vi "ramp autonomous.vi"() -> ()   [LabVIEW 2012, in "Omni2013.lvrbt"]
uses:
  Omni2013.lvrbt
  <vilib>/NXT/Hardware/Plugins/Tetrix 180 deg Servo/Tetrix180ServoAddress.ctl
  <vilib>/NXT/Hardware/Plugins/Tetrix DC Motor/TetrixDCMotorAddress.ctl
  <vilib>/NXT/HiTechnic/HiTechnic Controls/HiTechnic Port.ctl
  <vilib>/NXT/Block Support/NXT_InputPort.ctl
  <vilib>/NXT/Dual Mode Library/Waits/Wait_Num(msec).vi
  <vilib>/NXT/NXTIO Xnodes/NXTIONodeSubVIs/TETRIX IO Move Servos.vi
  <vilib>/NXT/NXTIO Xnodes/NXTIONodeSubVIs/TETRIX IO Move DC Motors.vi
  <vilib>/NXT/HiTechnic/HiTechnic Config/HiTechnic IRSeeker Mode1200Hz.vi
  <vilib>/NXT/HiTechnic/HiTechnic SubVIs/HiTechnic IRSeeker Sensor_AC dir.vi
  <vilib>/NXT/Dual Mode Library/Sensors/Sonar_cm.vi
  <vilib>/NXT/Dual Mode Library/Display/drawNumber.vi
  <vilib>/NXT/HiTechnic/HiTechnic Read/HiTechnic IRSeeker Sensor_DC all.vi
  <vilib>/NXT/NXTIO Xnodes/AddressXNode/NXTIOAddress.xnode
  <vilib>/NXT/NXTIO Xnodes/NXTIOXNode/NXTIO.xnode
  <vilib>/NXT/Subs/LVHSConnector.ctl
  <vilib>/NXT/LegoClasses/BrickReference/BrickReference.lvclass
panel:
  in  "Rotation":dbl
  in  "Translation L&R":dbl
  in  "Translation U&D":dbl
  in  "Initial Time":dbl
  out "Enabled":bool
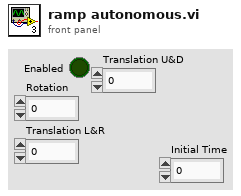
[diagram p1: front panel]
types:
  T1 = typedef "LVHSConnector.ctl" = refnum<class "BrickReference.lvclass">
  T2 = typedef "HiTechnic Port.ctl" = cluster{"Port":T3, "MUX Port":u8}
  T3 = typedef "NXT_InputPort.ctl" = u8
  T4 = typedef "TetrixDCMotorAddress.ctl" = i16
  T5 = cluster{"TetrixDCMotor":T4, "TetrixDCMotor 2":T4}
  T6 = cluster{"Direction (0-9)":i16, "Signal Strength (Array)":u8[]}
  T7 = typedef "Tetrix180ServoAddress.ctl" = i16
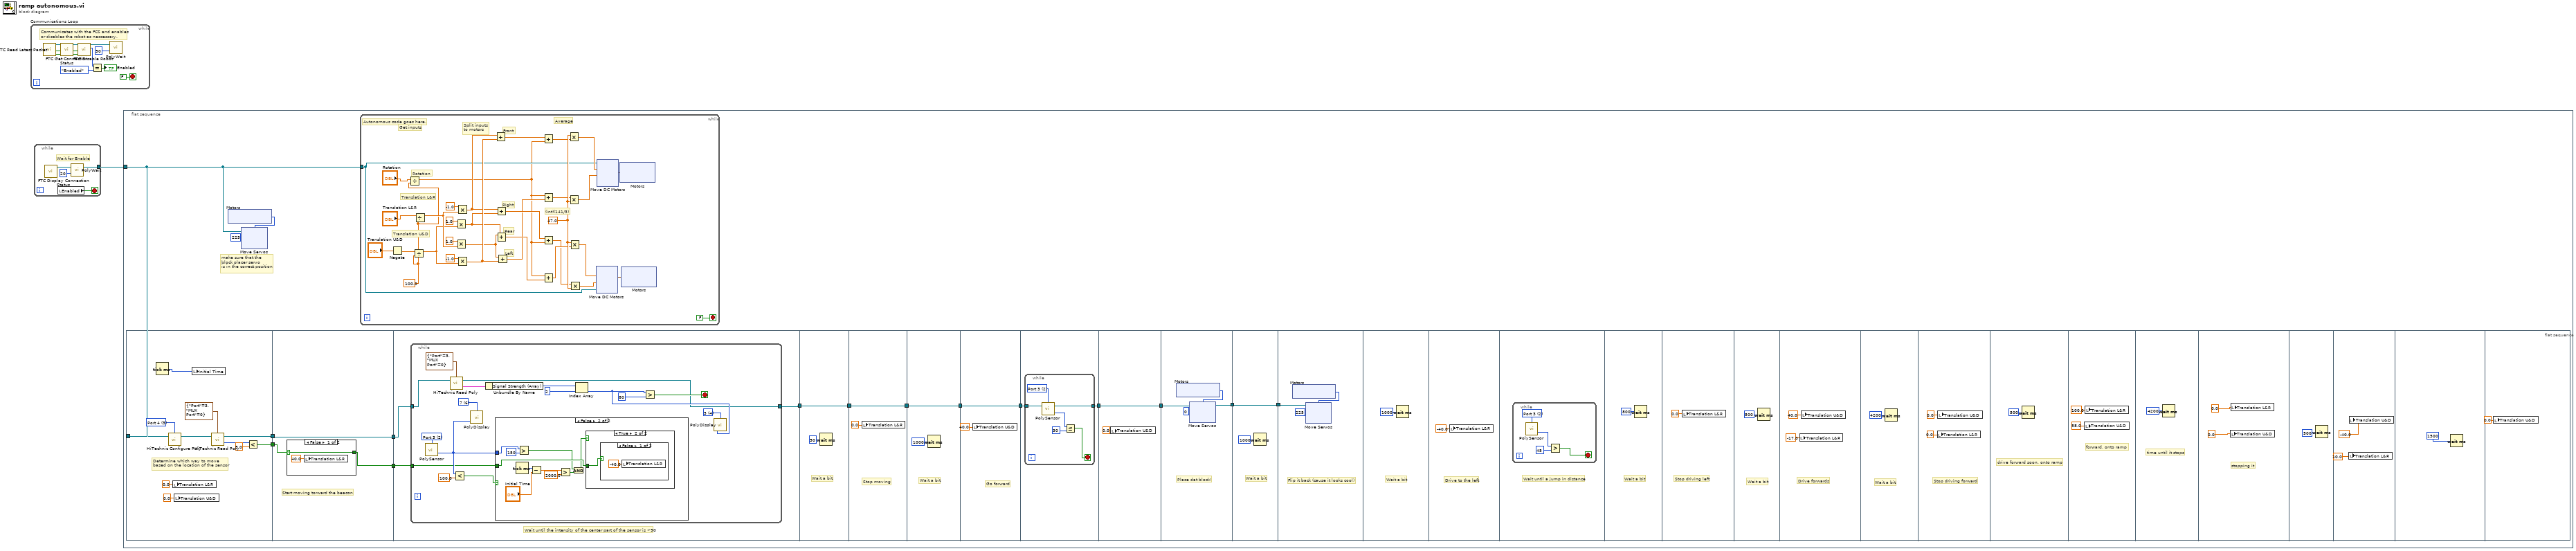
[diagram p0: block diagram]
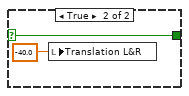
[diagram p2: hidden frame]
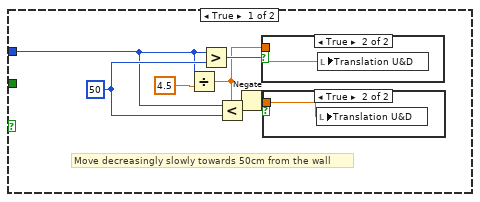
[diagram p3: hidden frame]
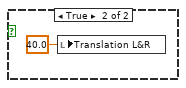
[diagram p7: hidden frame]
diagram:
  n1 = while "Communications Loop" {
    stop <- FALSE stop-if-true
    # "Communicates with the FCS and enables \nor disables the robot as neccessary."
    n2 = call <vilib>:"FTC Read Latest Packet.vi"() -> ("Packet Received?"=w11:bool, "Stopped?"=w10:bool, "NXT"=w13:T1)  [unwired: 6 in, 3 out]
    n3 = call <vilib>:"FTC Get Connection Status.vi"("Packet Received?"=w11, "Stopped?"=w10, "NXT"=w13) -> ("Online?"=w2:bool, "Stopped?"=w3:bool, "NXT"=w12:T1)  [unwired: 5 in]
    n4 = call <vilib>:"FTC Disable Robot.vi"("Online?"=w2, "Stopped?"=w3, "NXT"=w12) -> ("Enabled?"=w6:enum16{"Disabled", "Enabled"}, "NXT"=w8:T1)  [unwired: 3 in]
    n5 = Equal?(x=w6, y=enum16{"Disabled", "Enabled"}."Enabled") -> (x = y?=→"Enabled":bool)
    n6 = call-poly <vilib>:"PolyWait.vi"("Time (100 msec)"=u32 50 ("Time (msec)"), "NXT"=w8) -> ()  [unwired: 2 in, 1 out]
  }
  n7 = while {
    tunnel: [w15] -> w1
    stop <- w16 stop-if-true
    # "Wait for Enable"
    n8 = call <vilib>:"FTC Display Connection Status.vi"() -> ("NXT"=w14:T1)  [unwired: 11 in]
    n9 = local read "Enabled"() -> (w16:bool)
    n10 = call-poly <vilib>:"PolyWait.vi"("Time (100 msec)"=u32 20 ("Time (msec)"), "NXT"=w14) -> ("NXT"=w15:T1)  [unwired: 2 in]
  }
  n11 = flat-sequence {
    tunnel: w1 -> [w31]
    frame #0 {
      # "make sure that the \nblock placer servo \nis in the correct position"
      n12 = flat-sequence {
        tunnel: [w52] -> w20
        tunnel: [w51] -> w19
        tunnel: w31 -> [w43]
        tunnel: [w55] -> w28
        tunnel: w20 -> [w54]
        tunnel: w19 -> [w55]
        tunnel: [w53] -> w18
        tunnel: w28 -> [w62]
        tunnel: [w61] -> w30
        tunnel: w18 -> [w60]
        tunnel: w30 -> [w102]
        tunnel: [w102] -> w29
        tunnel: [w103] -> w27
        tunnel: w29 -> [w103]
        tunnel: [w106] -> w21
        tunnel: w27 -> [w106]
        tunnel: w21 -> [w108]
        tunnel: [w108] -> w26
        tunnel: w26 -> [w110]
        tunnel: [w109] -> w25
        tunnel: w25 -> [w118]
        tunnel: [w118] -> w24
        tunnel: w24 -> [w120]
        tunnel: [w119] -> w23
        tunnel: w23 -> [w132]
        tunnel: [w132] -> w22
        tunnel: w22 -> [w133]
        frame #0 {
          w46 = T3 3 items=["Port 1", "Port 2", "Port 3", "Port 4"] ("Port")
          # "Determine which way to move \nbased on the location of the sensor"
          n13 = Tick Count (ms)() -> (millisecond timer value=w42:u32)
          n14 = call-poly <vilib>:"HiTechnic Configure Poly.vi"("NXT"=w43, "Port"=w46) -> ("NXT"=w47:T1)  [unwired: 2 in]
          n15 = local write "Translation L&R"(0.0 ("Translation L&R")) -> ()
          n16 = local write "Translation U&D"(0.0 ("Translation U&D")) -> ()
          n17 = local write "Initial Time"(w42) -> ()
          n18 = call-poly <vilib>:"HiTechnic Read Poly.vi"("NXT"=w47, "Port/MUX"=T2 {"Port"=3, "MUX Port"=0}) -> ("Direction (0-9)"=w48:i16, "NXT"=w51:T1)  [unwired: 1 in]
          n19 = Less?(x=w48, y=5.0) -> (x < y?=w52:bool)
        }
        frame #1 {
          # "Start moving torward the beacon"
          n20 = case shown="False" w54 {
            selector: w54 -> [w56 w58]
            tunnel: [w56 w58] -> w53
            frame False {
              n21 = local write "Translation L&R"(40.0 ("Translation L&R")) -> ()
            }
            frame True {
              n22 = local write "Translation L&R"(-40.0 ("Translation L&R")) -> ()
            }
          }
        }
        frame #2 {
          # "Wait until the intensity of the center part of the sensor is >90"
          n23 = while {
            tunnel: w62 -> [w70]
            tunnel: [w68] -> w61
            tunnel: w60 -> [w63]
            stop <- w74 stop-if-true
            w67 = i16 6 items=["1", "2", "3", "4", "5", "6", "7", "8"] ("Line")
            w69 = T3 2 items=["Port 1", "Port 2", "Port 3", "Port 4"] ("Port (Port 4)")
            w73 = i16 4 items=["1", "2", "3", "4", "5", "6", "7", "8"] ("Line")
            n24 = call-poly <vilib>:"PolySensor.vi"("Port (Port 4)"=w69) -> ("Distance (cm)"=w65:i16)  [unwired: 2 in, 1 out]
            n25 = call-poly <vilib>:"HiTechnic Read Poly.vi"("NXT"=w70, "Port/MUX"=T2 {"Port"=3, "MUX Port"=0}) -> ("All Info"=w77:T6, "NXT"=w68:T1)  [unwired: 1 in]
            n26 = Less?(x=w65, y=100.0) -> (x < y?=w64:bool)
            n27 = call-poly <vilib>:"PolyDisplay.vi"("number"=w65, "Line"=w67) -> ()  [unwired: 2 in, 1 out]
            n28 = Unbundle By Name(w77) -> ("Signal Strength (Array)"=w76:u8[])
            n29 = case shown="False" w64 {
              tunnel: w65 -> [w81 w97]
              tunnel: w63 -> [_ w95]
              frame True {
                w83 = i16 50 ("y")
                # "Move decreasingly slowly towards 50cm from the wall"
                n30 = Divide(x=w81, y=4.5) -> (x/y=w80:dbl)
                n31 = Greater?(x=w81, y=w83) -> (0:w84:bool)
                n32 = Less?(x=w81, y=w83) -> (x < y?=w85:bool)
                n33 = Negate(x=w80) -> (-x=w79:dbl)
                n34 = case shown="True" w84 {
                  tunnel: w80 -> [_ w86]
                  frame False {
                  }
                  frame True {
                    n35 = local write "Translation U&D"(w86) -> ()
                  }
                }
                n36 = case shown="True" w85 {
                  tunnel: w79 -> [_ w87]
                  frame False {
                  }
                  frame True {
                    n37 = local write "Translation U&D"(w87) -> ()
                  }
                }
              }
              frame False {
                n38 = Tick Count (ms)() -> (millisecond timer value=w94:u32)
                n39 = Greater?(x=w97, y=i16 150) -> (0:w89:bool)
                n40 = Subtract(x=w94, y="Initial Time") -> (x-y=w92:dbl)
                n41 = Greater?(x=w92, y=2000.0) -> (0:w88:bool)
                n42 = And(x=w89, y=w88) -> (x .and. y?=w90:bool)
                n43 = case shown="True" w90 {
                  tunnel: w95 -> [_ w98]
                  frame False {
                  }
                  frame True {
                    n44 = case shown="False" w98 {
                      frame False {
                        n45 = local write "Translation L&R"(-40.0 ("Translation L&R")) -> ()
                      }
                      frame True {
                        n46 = local write "Translation L&R"(40.0 ("Translation L&R")) -> ()
                      }
                    }
                  }
                }
              }
            }
            n47 = Index Array(array=w76, index=2) -> (element=w72:u8)
            n48 = Greater?(x=w72, y=u8 80) -> (0:w74:bool)
            n49 = call-poly <vilib>:"PolyDisplay.vi"("number"=w72, "Line"=w73) -> ()  [unwired: 2 in, 1 out]
          }
        }
        frame #3 {
          # "Wait a bit"
          n50 = Wait (ms)(milliseconds to wait=u32 50) -> ()  [unwired: 1 out]
        }
        frame #4 {
          # "Stop moving"
          n51 = local write "Translation L&R"(0.0 ("Translation L&R")) -> ()
        }
        frame #5 {
          # "Wait a bit"
          n52 = Wait (ms)(milliseconds to wait=u32 1000) -> ()  [unwired: 1 out]
        }
        frame #6 {
          # "Go forward"
          n53 = local write "Translation U&D"(40.0 ("Translation U&D")) -> ()
        }
        frame #7 {
          n54 = while {
            tunnel: w110 -> [w113]
            tunnel: [w112] -> w109
            stop <- w114 stop-if-true
            w111 = T3 2 items=["Port 1", "Port 2", "Port 3", "Port 4"] ("Port (Port 4)")
            n55 = call-poly <vilib>:"PolySensor.vi"("NXT"=w113, "Port (Port 4)"=w111) -> ("Distance (cm)"=w116:i16, "NXT"=w112:T1)  [unwired: 1 in]
            n56 = Less Or Equal?(x=w116, y=i16 30) -> (x <= y?=w114:bool)
          }
        }
        frame #8 {
          n57 = local write "Translation U&D"(0.0 ("Translation U&D")) -> ()
        }
        frame #9 {
          # "Place dat block!"
          n58 = xnode "Motors"() -> ("Motor"=w122:T7)
          n59 = xnode "Move Servos"("Position 1"=u8 0, "Servos"=w122, "NXT"=w120) -> ("NXT"=w119:T1)
        }
        frame #10 {
          # "Wait a bit"
          n60 = Wait (ms)(milliseconds to wait=u32 1000) -> ()  [unwired: 1 out]
        }
        frame #11 {
          # "Flip it back (cause it looks cool)"
          n61 = xnode "Motors"() -> ("Motor"=w135:T7)
          n62 = xnode "Move Servos"("Position 1"=u8 225, "Servos"=w135, "NXT"=w133) -> ()  [unwired: 1 out]
        }
        frame #12 {
          # "Wait a bit"
          n63 = Wait (ms)(milliseconds to wait=u32 1000) -> ()  [unwired: 1 out]
        }
        frame #13 {
          # "Drive to the left"
          n64 = local write "Translation L&R"(-40.0 ("Translation L&R")) -> ()
        }
        frame #14 {
          # "Wait until a jump in distance"
          n65 = while {
            stop <- w147 stop-if-true
            w149 = T3 2 items=["Port 1", "Port 2", "Port 3", "Port 4"] ("Port (Port 4)")
            n66 = call-poly <vilib>:"PolySensor.vi"("Port (Port 4)"=w149) -> ("Distance (cm)"=w146:i16)  [unwired: 2 in, 1 out]
            n67 = Greater?(x=w146, y=i16 45) -> (0:w147:bool)
          }
        }
        frame #15 {
          # "Wait a bit"
          n68 = Wait (ms)(milliseconds to wait=u32 800) -> ()  [unwired: 1 out]
        }
        frame #16 {
          # "Stop driving left"
          n69 = local write "Translation L&R"(0.0 ("Translation L&R")) -> ()
        }
        frame #17 {
          # "Wait a bit"
          n70 = Wait (ms)(milliseconds to wait=u32 500) -> ()  [unwired: 1 out]
        }
        frame #18 {
          # "Drive forwards"
          n71 = local write "Translation L&R"(-17.0 ("Translation L&R")) -> ()
          n72 = local write "Translation U&D"(40.0 ("Translation U&D")) -> ()
        }
        frame #19 {
          # "Wait a bit"
          n73 = Wait (ms)(milliseconds to wait=u32 4200) -> ()  [unwired: 1 out]
        }
        frame #20 {
          # "Stop driving forward"
          n74 = local write "Translation L&R"(0.0 ("Translation L&R")) -> ()
          n75 = local write "Translation U&D"(0.0 ("Translation U&D")) -> ()
        }
        frame #21 {
          # "drive forward soon, onto ramp"
          n76 = Wait (ms)(milliseconds to wait=u32 500) -> ()  [unwired: 1 out]
        }
        frame #22 {
          # "forward, onto ramp"
          n77 = local write "Translation U&D"(58.0 ("Translation U&D")) -> ()
          n78 = local write "Translation L&R"(100.0 ("Translation L&R")) -> ()
        }
        frame #23 {
          # "time until it stops"
          n79 = Wait (ms)(milliseconds to wait=u32 4200) -> ()  [unwired: 1 out]
        }
        frame #24 {
          # "stopping it"
          n80 = local write "Translation U&D"(0.0 ("Translation U&D")) -> ()
          n81 = local write "Translation L&R"(0.0 ("Translation L&R")) -> ()
        }
        frame #25 {
          n82 = Wait (ms)(milliseconds to wait=u32 500 ("millisecond timer value")) -> ()  [unwired: 1 out]
        }
        frame #26 {
          n83 = local write "Translation L&R"(10.0 ("Translation L&R")) -> ()
          n84 = local write "Translation U&D"(-40.0 ("Translation U&D")) -> ()
        }
        frame #27 {
          n85 = Wait (ms)(milliseconds to wait=u32 1500 ("millisecond timer value")) -> ()  [unwired: 1 out]
        }
        frame #28 {
          n86 = local write "Translation U&D"(0.0 ("Translation U&D")) -> ()
        }
      }
      n87 = xnode "Motors"() -> ("Motor"=w33:T7)
      n88 = xnode "Move Servos"("Position 1"=u8 225, "Servos"=w33, "NXT"=w31) -> ()  [unwired: 1 out]
      n89 = while {
        tunnel: w31 -> [w174]
        stop <- FALSE stop-if-true
        w170 = 100.0 ("y")
        w201 = 47.0 ("y")
        # "Average"
        # "Left"
        # "Rear"
        # "Right"
        # "Front"
        # "(int)(141/3)"
        # "Split inputs to motors"
        # "Get inputs"
        # "Translation U&D"
        # "Rotation"
        # "Translation L&R"
        # "Autonomous code goes here."
        n90 = Negate(x="Translation U&D") -> (-x=w169:dbl)
        n91 = Divide(x="Rotation", y=w170) -> (x/y=w171:dbl)
        n92 = Divide(x=w169, y=w170) -> (x/y=w172:dbl)
        n93 = Divide(x="Translation L&R", y=w170) -> (x/y=w173:dbl)
        n94 = Multiply(x=1.0, y=w172) -> (x*y=w195:dbl)
        n95 = Multiply(x=1.0, y=w173) -> (x*y=w184:dbl)
        n96 = Multiply(x=-1.0, y=w173) -> (x*y=w183:dbl)
        n97 = Multiply(x=-1.0, y=w172) -> (x*y=w196:dbl)
        n98 = Add(x=w183, y=w196) -> (x+y=w180:dbl)
        n99 = Add(x=w183, y=w195) -> (x+y=w182:dbl)
        n100 = Add(x=w184, y=w195) -> (x+y=w179:dbl)
        n101 = Add(x=w184, y=w196) -> (x+y=w181:dbl)
        n102 = Add(x=w180, y=w171) -> (x+y=w199:dbl)
        n103 = Add(x=w171, y=w181) -> (x+y=w198:dbl)
        n104 = Add(x=w182, y=w171) -> (x+y=w197:dbl)
        n105 = Add(x=w171, y=w179) -> (x+y=w200:dbl)
        n106 = Multiply(x=w201, y=w199) -> (x*y=w190:dbl)
        n107 = Multiply(x=w198, y=w201) -> (x*y=w191:dbl)
        n108 = Multiply(x=w201, y=w200) -> (x*y=w194:dbl)
        n109 = Multiply(x=w197, y=w201) -> (x*y=w193:dbl)
        n110 = xnode "Motors"() -> ("Motor"=w189:cluster{"TetrixDCMotor":T4, "TetrixDCMotor":T4})
        n111 = xnode "Move DC Motors"("Power/Speed 2"=w191, "Power/Speed 1"=w190, "Motors"=w189, "NXT"=w174) -> ()  [unwired: 1 out]
        n112 = xnode "Motors"() -> ("Motor"=w192:cluster{"TetrixDCMotor":T4, "TetrixDCMotor":T4})
        n113 = xnode "Move DC Motors"("Power/Speed 2"=w193, "Power/Speed 1"=w194, "Motors"=w192, "NXT"=w174) -> ()  [unwired: 1 out]
      }
    }
  }
